vi "online(server1st).vi"() -> ()   [LabVIEW 2022 SP3]
panel:
  in  "OK Button":bool
  in  "stop":bool
  out "isMyTurn?":bool
  in  "value":i32[][](array[numeric])
  # "與online(client1st)成對，為正式使用於黑白棋前的測試，確認可以雙方輪流作為server送資料/client接收資料\n此為先作為server者，使用方式為修改陣列裡的值並按ok，再傳出後到收到前ok按鈕會隱藏"
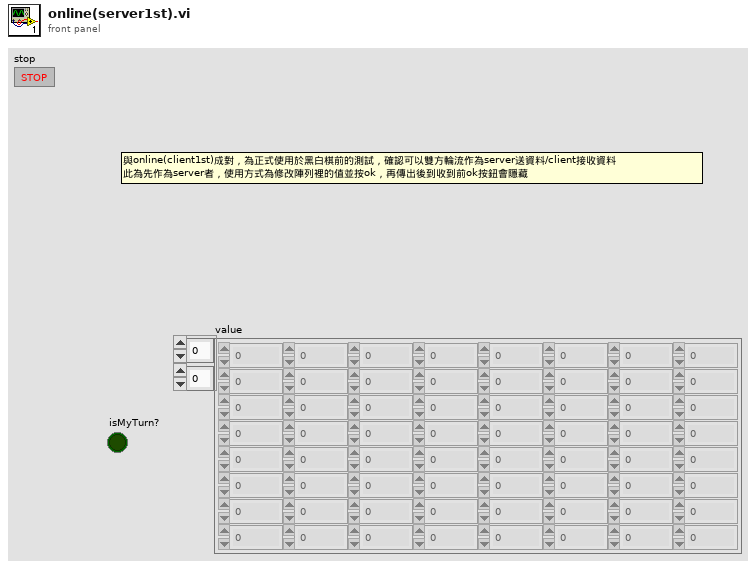
[diagram p1: front panel]
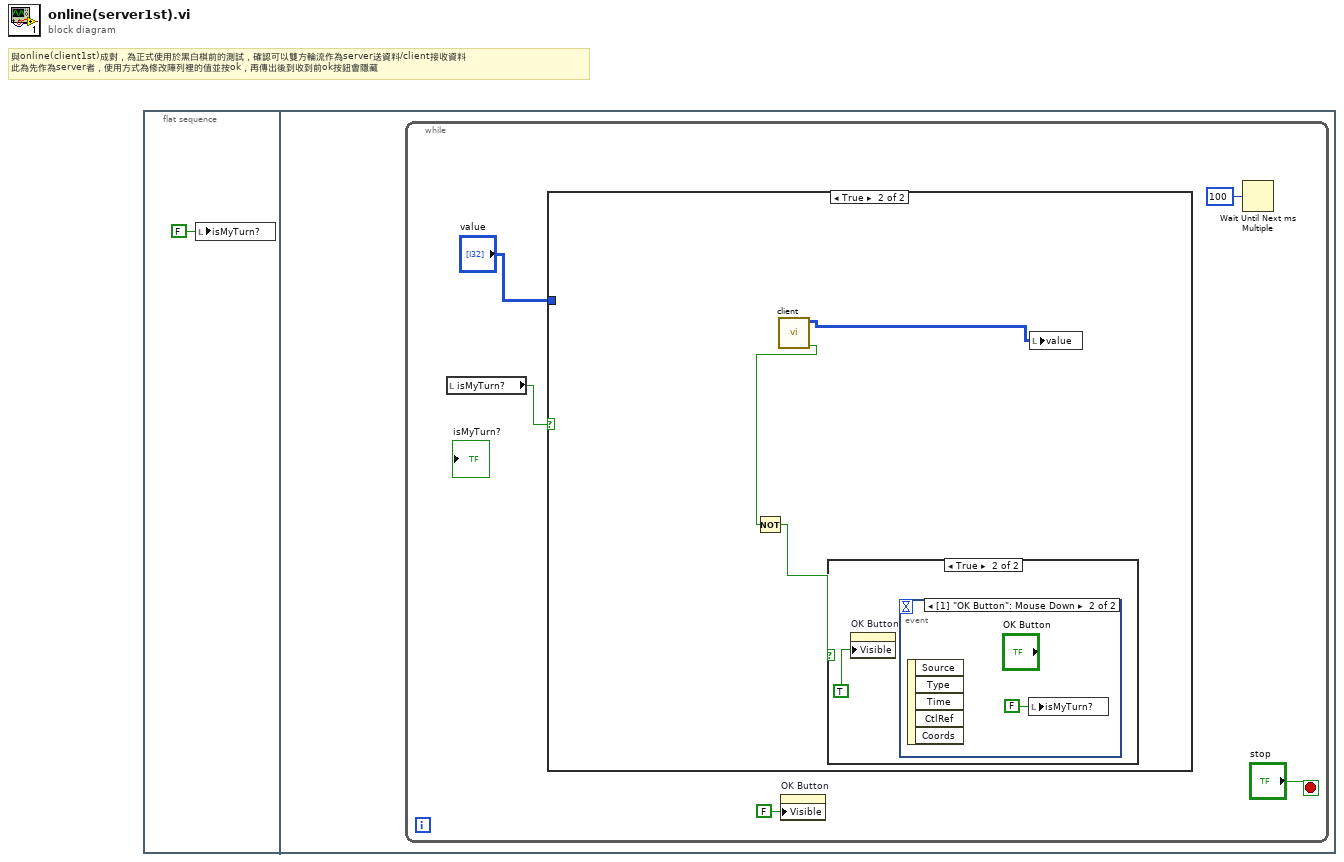
[diagram p0: block diagram]
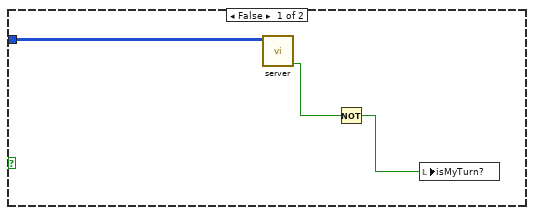
[diagram p2: hidden frame]
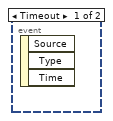
[diagram p4: hidden frame]
diagram:
  # "與online(client1st)成對，為正式使用於黑白棋前的測試，確認可以雙方輪流作為server送資料/client接收資料\n此為先作為server者，使用方式為修改陣列裡的值並按ok，再傳出後到收到前ok按鈕會隱藏"
  n1 = flat-sequence {
    frame #0 {
      n2 = local write "isMyTurn?"(FALSE ("isMyTurn?")) -> ()
    }
    frame #1 {
      n3 = while {
        stop <- "stop" stop-if-true
        n4 = local read "isMyTurn?"() -> (w4:bool)
        n5 = case shown="True" w4 {
          tunnel: "value" -> [w9 _]
          frame False {
            n6 = call "server.vi"("array"=w9) -> ("error"=w8:bool)  [unwired: 10 in]
            n7 = Not(x=w8) -> (.not. x?=w7:bool)
            n8 = local write "isMyTurn?"(w7) -> ()
          }
          frame True {
            n9 = call "client.vi"() -> ("error"=w11:bool, "value"=w12:i32[][])  [unwired: 10 in]
            n10 = Not(x=w11) -> (.not. x?=w10:bool)
            n11 = case shown="True" w10 {
              frame False {
              }
              frame True {
                n12 = property on="OK Button" class="Bool (strict)"("Visible"=TRUE) -> ()  [unwired: 2 in, 2 out]
                n13 = event shown="[1] \"OK Button\": Mouse Down" {
                  selector: _ -> [_ _]
                  dyn-events: _ -> [_ _]
                  timeout: _ -> [_ _]
                  event Timeout {
                    n14 = event-data() -> ()  [unwired: 1 in, 3 out]
                  }
                  event "OK Button": Mouse Down {
                    n15 = event-data() -> ()  [unwired: 1 in, 5 out]
                    n16 = local write "isMyTurn?"(FALSE ("isMyTurn?")) -> ()
                  }
                }
              }
            }
            n17 = local write "value"(w12) -> ()
          }
        }
        n18 = property on="OK Button" class="Bool (strict)"("Visible"=FALSE) -> ()  [unwired: 2 in, 2 out]
        n19 = Wait Until Next ms Multiple(millisecond multiple=u32 100) -> ()  [unwired: 1 out]
      }
    }
  }
